vi "Command (write) - FL.vi"(7 "timeout ms (100)":i32=100, 8 "error in (no error)":errorcluster, 9 "Distance":i32, 10 "IP":string, 11 "connection ID in":refnum<k16>) -> (0 "error out":errorcluster, 3 "connection ID out":refnum<k16>)   [LabVIEW 2016, in "SMD-7615.lvlib" / "eSCL.lvlib"]
doc: "FL - Feed to Length\nExecutes a relative move command. Move distance and direction come from the last DI command. Speed, accel and decel are from the VE, AC and DE commands, respectively. Executing the FL command with no\nparameter initiates a feed to length move that uses the last DI command for direction and distance. Executing the FL command with a parameter uses the parameter settings for direction and distance without changing the DI command."
uses:
  eSCL.lvlib
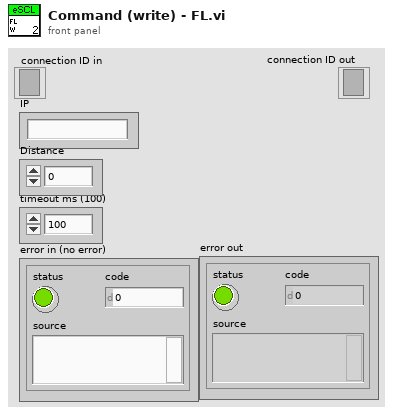
[diagram p1: front panel]
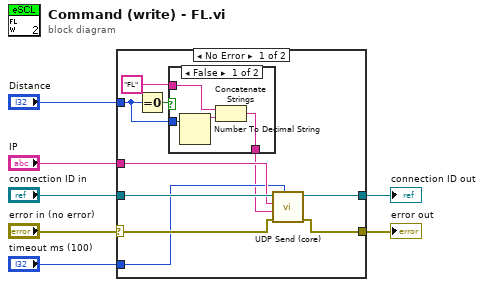
[diagram p0: block diagram]
diagram:
  n1 = case shown="No Error" "error in (no error)" {
    selector: "error in (no error)" -> [w17 w23]
    tunnel: "connection ID in" -> [w16 w24]
    tunnel: [w12 w24] -> w5
    tunnel: [w11 w23] -> w4
    tunnel: "IP" -> [w15 _]
    tunnel: "timeout ms (100)" -> [w14 _]
    tunnel: "Distance" -> [w9 _]
    frame No Error {
      n2 = Equal To 0?(x=w9) -> (x = 0?=w8:bool)
      n3 = case shown="False" w8 {
        tunnel: "FL" ("Data") -> [w21 w22]
        tunnel: [w20 w22] -> w10
        tunnel: w9 -> [w19 _]
        frame False {
          n4 = Number To Decimal String(number=w19) -> (decimal integer string=w18:string)  [unwired: 1 in]
          n5 = Concatenate Strings(w21, w18) -> (w20:string)
        }
        frame True {
        }
      }
      n6 = call "UDP Send (core).vi"("timeout ms (100)"=w14, "error in (no error)"=w17, "Data"=w10, "IP"=w15, "connection ID in"=w16) -> ("error out"=w11:errorcluster, "connection ID out"=w12:refnum<k16>)  [unwired: 5 in]
    }
    frame Error {
    }
  }
  "connection ID out" <- w5
  "error out" <- w4
